vi "Proceso.vi"() -> ()   [LabVIEW 2019, in "Class 2.lvclass"]
uses:
  Class 2.lvclass
  Class 2.lvclass/Class 2.ctl
panel:
  in  "stop":bool
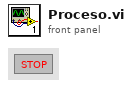
[diagram p1: front panel]
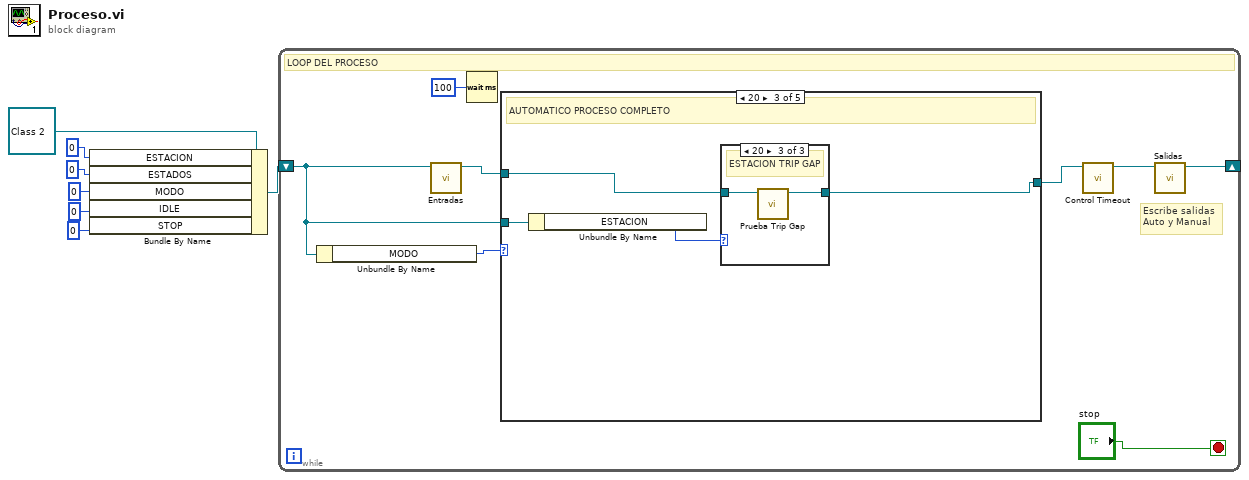
[diagram p0: block diagram]
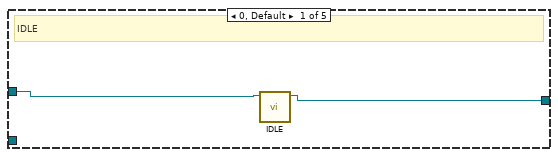
[diagram p2: hidden frame]
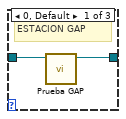
[diagram p4: hidden frame]
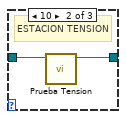
[diagram p5: hidden frame]
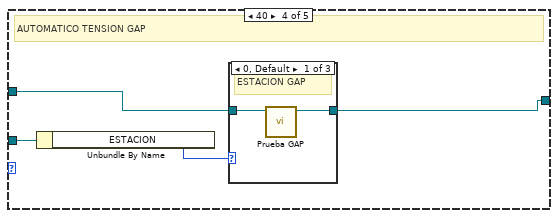
[diagram p6: hidden frame]
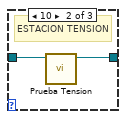
[diagram p7: hidden frame]
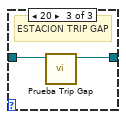
[diagram p8: hidden frame]
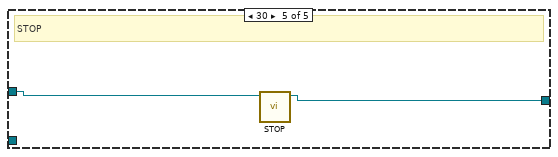
[diagram p9: hidden frame]
diagram:
  n1 = Bundle By Name(cluster=refnum<class "Class 2.lvclass"> refnum ("Class 2.lvclass"), "ESTACION"=0 ("State"), "ESTADOS"=i16 0 ("SubState"), "MODO"=i16 0 ("MAQ DE ESTADOS.MODO"), "IDLE"=i16 0 ("MAQ DE ESTADOS.IDLE"), "STOP"=i16 0 ("MAQ DE ESTADOS.STOP")) -> (w4:refnum<class "Class 2.lvclass">)
  n2 = while {
    shift-right: [w13] -> _
    shift-left: w4 -> [w12]
    stop <- "stop" stop-if-true
    # "Escribe salidas\nAuto y Manual"
    # "LOOP DEL PROCESO"
    n3 = Unbundle By Name(w12) -> ("MODO"=w10:i16)
    n4 = call "Entradas.vi"("Class 2.lvclass"=w12) -> ("Class 2.lvclass 2"=w14:refnum<class "Class 2.lvclass">)  [unwired: 10 in]
    n5 = Wait (ms)(milliseconds to wait=u32 100) -> ()  [unwired: 1 out]
    n6 = case shown="20" w10 {
      tunnel: w12 -> [_ _ w21 w31 _]
      tunnel: w14 -> [w17 w18 w20 w30 w40]
      tunnel: [w16 w18 w19 w29 w39] -> w9
      frame 0, Default {
        # "IDLE"
        n7 = call "IDLE.vi"("Class 2.lvclass"=w17) -> ("Class 2.lvclass 2"=w16:refnum<class "Class 2.lvclass">)  [unwired: 10 in]
      }
      frame 10 {
        # "LOGGING"
      }
      frame 20 {
        # "AUTOMATICO PROCESO COMPLETO"
        n8 = Unbundle By Name(w21) -> ("ESTACION"=w22:i32)
        n9 = case shown="20" w22 {
          tunnel: w20 -> [w24 w26 w28]
          tunnel: [w23 w25 w27] -> w19
          frame 0, Default {
            # "ESTACION GAP"
            n10 = call "Prueba GAP.vi"("Class 2.lvclass"=w24) -> ("Class 2.lvclass 2"=w23:refnum<class "Class 2.lvclass">)  [unwired: 10 in]
          }
          frame 10 {
            # "ESTACION TENSION"
            n11 = call "Prueba Tension.vi"("Class 2.lvclass"=w26) -> ("Class 2.lvclass 2"=w25:refnum<class "Class 2.lvclass">)  [unwired: 10 in]
          }
          frame 20 {
            # "ESTACION TRIP GAP"
            n12 = call "Prueba Trip Gap.vi"("Class 2.lvclass"=w28) -> ("Class 2.lvclass 2"=w27:refnum<class "Class 2.lvclass">)  [unwired: 10 in]
          }
        }
      }
      frame 40 {
        # "AUTOMATICO TENSION GAP"
        n13 = Unbundle By Name(w31) -> ("ESTACION"=w32:i32)
        n14 = case shown="0, Default" w32 {
          tunnel: w30 -> [w34 w36 w38]
          tunnel: [w33 w35 w37] -> w29
          frame 0, Default {
            # "ESTACION GAP"
            n15 = call "Prueba GAP.vi"("Class 2.lvclass"=w34) -> ("Class 2.lvclass 2"=w33:refnum<class "Class 2.lvclass">)  [unwired: 10 in]
          }
          frame 10 {
            # "ESTACION TENSION"
            n16 = call "Prueba Tension.vi"("Class 2.lvclass"=w36) -> ("Class 2.lvclass 2"=w35:refnum<class "Class 2.lvclass">)  [unwired: 10 in]
          }
          frame 20 {
            # "ESTACION TRIP GAP"
            n17 = call "Prueba Trip Gap.vi"("Class 2.lvclass"=w38) -> ("Class 2.lvclass 2"=w37:refnum<class "Class 2.lvclass">)  [unwired: 10 in]
          }
        }
      }
      frame 30 {
        # "STOP"
        n18 = call "STOP.vi"("Class 2.lvclass"=w40) -> ("Class 2.lvclass 2"=w39:refnum<class "Class 2.lvclass">)  [unwired: 10 in]
      }
    }
    n19 = call "Control Timeout.vi"("Class 2 in"=w9) -> ("Class 2 out"=w8:refnum<class "Class 2.lvclass">)  [unwired: 10 in]
    n20 = call "Salidas.vi"("Class 2.lvclass"=w8) -> ("Class 2.lvclass 2"=w13:refnum<class "Class 2.lvclass">)  [unwired: 10 in]
  }
